vi "hysteresis.vi"() -> ()   [LabVIEW 2018]
uses:
  <vilib>/Utility/file.llb/Read Delimited Spreadsheet (DBL).vi
panel:
  out "Prepared by \nthe project":string
  out "H percentage":dbl
  out "O increasing min":dbl
  out "Oncrieasing max":dbl
  out "Hmax":dbl
  out "H":dbl[](array[numeric])
  out "out decreasing":dbl[](array[numeric])
  out "out increasing":dbl[](array[numeric])
  out "in (kg)":sgl[](array[numeric])
  in  "Enter The Number \nof Measurements":i32
  in  "Measurement file \nwith extension Txt":path
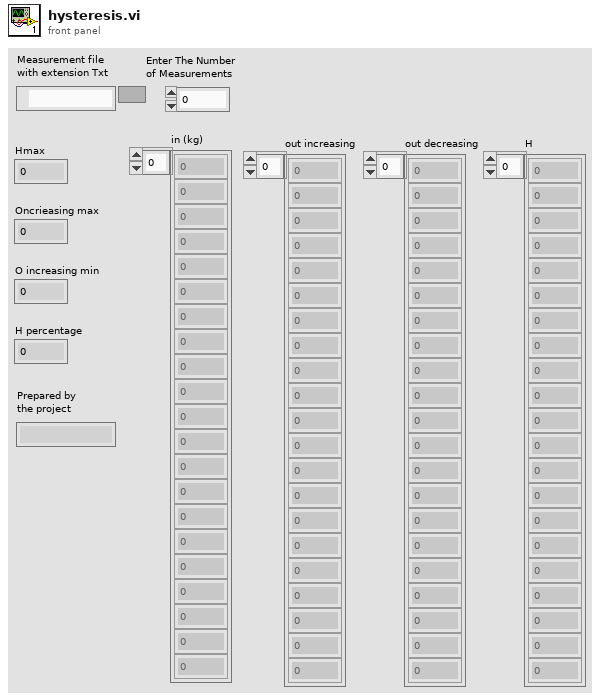
[diagram p1: front panel]
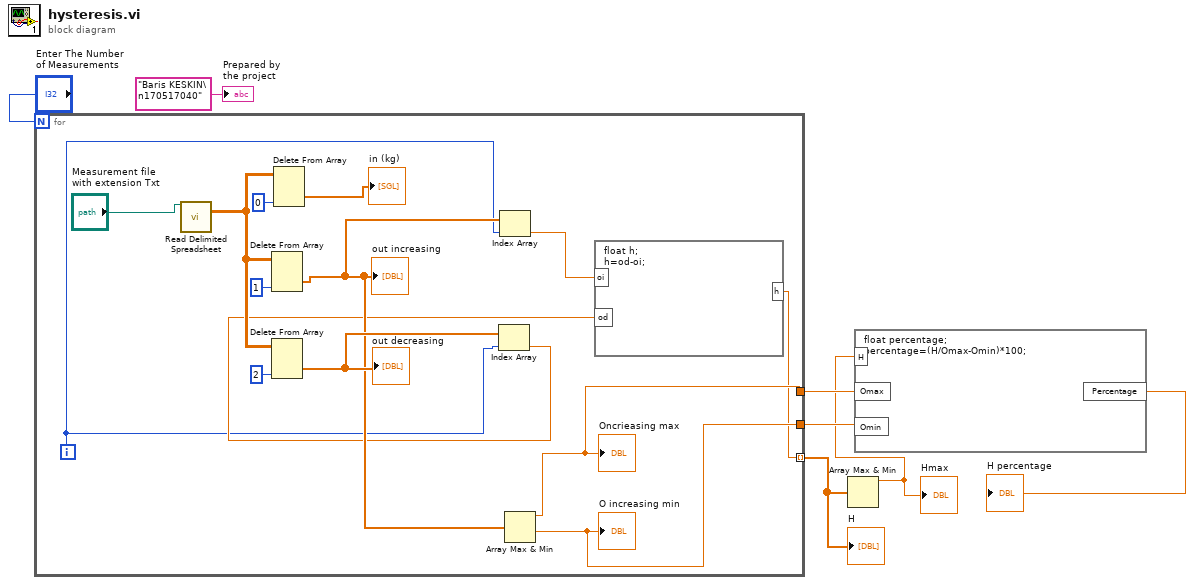
[diagram p0: block diagram]
diagram:
  n1 = for {
    N: "Enter The Number \nof Measurements" -> [_]
    tunnel: [w13] -> w5
    tunnel: [w12] -> w6
    tunnel: [w8] -> w3 mode=indexing
    i -> [w9]
    n2 = call-poly <vilib>:"Read Delimited Spreadsheet.vi"("file path (dialog if empty)"="Measurement file \nwith extension Txt") -> ("all rows"=w20:dbl[][])  [unwired: 9 in, 5 out]
    n3 = Delete From Array(array=w20, index (col)=1 ("disabled index (col)")) -> (deleted portion=w14:dbl[])  [unwired: 2 in, 1 out]
    "out increasing" <- w14
    n4 = Delete From Array(array=w20, index (col)=2 ("disabled index (col)")) -> (deleted portion=w17:dbl[])  [unwired: 2 in, 1 out]
    "out decreasing" <- w17
    n5 = Delete From Array(array=w20, index (col)=0 ("disabled index (col)")) -> (deleted portion=→"in (kg)":dbl[])  [unwired: 2 in, 1 out]
    n6 = Index Array(array=w17, index=w9) -> (element=w10:dbl)
    n7 = Index Array(array=w14, index=w9) -> (element=w11:dbl)
    n8 = Array Max & Min(array=w14) -> (max value=w12:dbl, min value=w13:dbl)  [unwired: 2 out]
    "Oncrieasing max" <- w12
    "O increasing min" <- w13
    n9 = formula code="float h;\nh=od-oi;"("oi"=w11, "od"=w10) -> ("h"=w8:dbl)
  }
  "H" <- w3
  n10 = Array Max & Min(array=w3) -> (max value=w2:dbl)  [unwired: 3 out]
  "Hmax" <- w2
  n11 = formula code="float percentage;\npercentage=(H/Omax-Omin)*100;"("H"=w2, "Omax"=w6, "Omin"=w5) -> ("Percentage"=→"H percentage":dbl)
  "Prepared by \nthe project" <- "Baris KESKIN\n170517040"
